vi "Add Timestamp to File and Directory.vi"(2 "File Path":path) -> (0 "appended path":path)   [LabVIEW 2009]
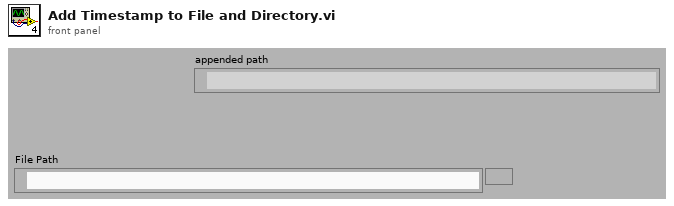
[diagram p1: front panel]
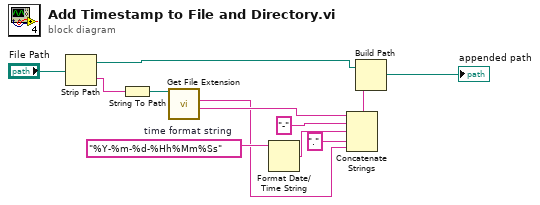
[diagram p0: block diagram]
diagram:
  w10 = "%Y-%m-%d-%Hh%Mm%Ss"  # time format string
  n1 = Strip Path(path="File Path") -> (stripped path=w3:path, name=w1:string)
  n2 = String To Path(string=w1) -> (path=w2:path)
  n3 = call <vilib>:"Get File Extension.vi"("file"=w2) -> ("filename without extension"=w7:string, "lowercase file extension"=w5:string)  [unwired: 7 in, 2 out]
  n4 = Format Date/Time String(time format string (%c)=w10) -> (date/time string=w11:string)  [unwired: 2 in]
  n5 = Concatenate Strings(w7, "-" ("string"), w11, "." ("string"), w5) -> (w9:string)
  n6 = Build Path(base path=w3, name or relative path=w9) -> (appended path=→"appended path":path)
